vi "LEBITplc.ProcCases.vi"(0 "i ref in":refnum<vi>, 1 "selector":string, 2 "Data":T1, 3 "call cluster":T2={"Object"="", "Selector"="", "CallType"=enum."synchronous", "Async Object"="", "Async Selector"="", "Data Descriptor"="", "Data"=[], "Error #"=0, "Expire"=0}, 5 "error in (no error)":errorcluster) -> (14 "i ref out":refnum<vi>, 17 "answer cluster":T2={"Object"="", "Selector"="", "CallType"=enum."synchronous", "Async Object"="", "Async Selector"="", "Data Descriptor"="", "Data"=[], "Error #"=0, "Expire"=0}, 19 "error out":errorcluster)   [LabVIEW 2014, in "LEBITplc.lvlib"]
doc: "This method is called by a process from within the default case in the event loop. The methods of a class that are linked to events will be called from THIS method. Add your code here."
uses:
  LEBITplc.lvlib
  CS_Core/CSSystem/CoreDefs/CoreDefs.call_type.ctl
  CS_Core/BaseProcess/BaseProcess.descriptor string definition.ctl
  CS_Core/CSSystem/CoreDefs/CoreDefs.rawDataType.ctl
  CS_Core/CSSystem/CoreDefs/CoreDefs.error_severity.ctl
  CS_Core/CSSystem/CoreDefs/CoreDefs.error_type.ctl
  CS_Core/CSSystem/CoreLib/CoreLib.byte array 2 short.vi
  CS_Core/CSSystem/CoreLib/CoreLib.byte array 2 double.vi
  CS_Core/CSSystem/CoreLib/CoreLib.byte array 2 string.vi
  CS_Core/CSSystem/CoreLib/CoreLib.string 2 byte array.vi
  CS_Core/BaseProcess/BaseProcess.lvlib
  CS_Core/CSSystem/CoreLib/CoreLib.lvlib
  CS_Core/CAEObj/CAEObj.lvlib
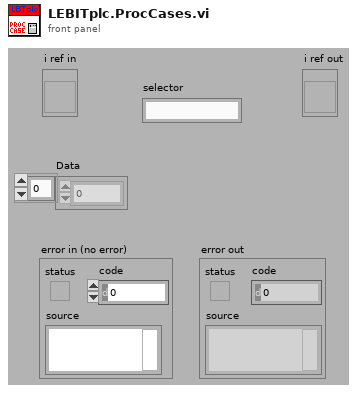
[diagram p1: front panel]
types:
  T1 = typedef "CoreDefs.rawDataType.ctl" = i8[]
  T2 = typedef "CoreDefs.call_type.ctl" = cluster{"Object":string, "Selector":string, "CallType":enum16{"simple", "synchronous", "asynchronous"}, "Async Object":string, "Async Selector":string, "Data Descriptor":T3, "Data":T1, "Error #":i32, "Expire":u32}
  T3 = typedef "BaseProcess.lvlib/BaseProcess.descriptor string definition.ctl" = string
  T4 = typedef "CoreDefs.error_type.ctl" = enum16{"no error", "can't load process", "can't unload process", "process does not exist", "can't install process", "can't remove process", "unknown function", "time out", "can't execute function", "duplicate queue name", "super not found", "caller queue invalid", "can't ping process", "unknown error", "VISA Error", "VISA timeout", "GPIB timeout", "GPIB error", "communication error", "data type mismatch", "can't read data from OPC server", "can't write data to OPC server", "OET error", "function not implemented", "process already exists", "invalid Shared Variable name", "error writing Shared Variable", "error reading Shared Variable", "invalid client name", "corrupt database", "unknown class", "call not authorized", "parameter out of range", "OET timeout: can't get data to modify", "invalid queue name", "requested operation incompatible with current state", "event undefined", "event disabled", "state undefined", "caller is not a friend", "EventBuilder: bad eventID", "EventBuilder: no DAQ devices", "a thread must not stop itself", "UNUSED ELEMENT4", "DiscArchiver: eventData incomplete", "DiscArchiver: eventData does not belong to run", "DiscArchiver: can't open file", "DiscArchiver: can't write to file", "DiscArchiver: available disc space low", "can't acquire semaphore", "error reading data from database", "notifier object is not existing", "can't register process", "can't unregister process", "illegal event type", "object disabled", "object already exists", "can't change state", "Instrument not found", "no connection to remote node", "invalid reference", "N/A", "UNUSED ELEMENT 1", "element not found", "illegal TCP/IP connection detected", "object does not exist", "invalid access ID", "unknown CS system", "invalid privilige", "unsupported data type", "unsupported server type", "IO server already exists", "Shared Variable already exists"}
  T5 = typedef "CoreDefs.error_severity.ctl" = enum16{"undefined", "information", "warning", "error", "fatal"}
  T6 = typedef "LEBITplc.lvlib/LEBITplc.i attribute.ctl" = cluster{"LLFLocation":string, "SetFileLocation":string, "nickNames":string[], "setValuePLCServiceID":i32[], "GUIServiceID":i32[], "monValuePLC":string[], "SetValueServiceID":i32[], "MonValueServiceID":i32[], "SetValue":dbl[][], "SetValueMin":dbl[], "SetValueMax":dbl[], "SetValueInfoServiceID":i32[], "GUINames":string[], "ListOfBases":string[], "Scale":dbl[], "Offset":dbl[], "setValuePLC":string[], "BaseName":string[], "ScaleServiceID":i32[], "OffsetServiceID":i32[], "AllPLCValues":string[], "CondSpecialArray":string[][], "CondSpecialIndex":i32[], "CondSpecialMonValue":dbl[], "RecentlyChanged":i32[], "SetFileLocationID":i32, "Dependent-Monitors":string[][], "LastLoadedFiles":string[], "IonGuideCalibLocation":string, "Monitor Dependent":string[], "Special":string[], "PLC?":bool[], "Start Date":string, "ListOfBasesServiceID":i32, "SETRA VISA resource":refnum<visa-resource-name>}
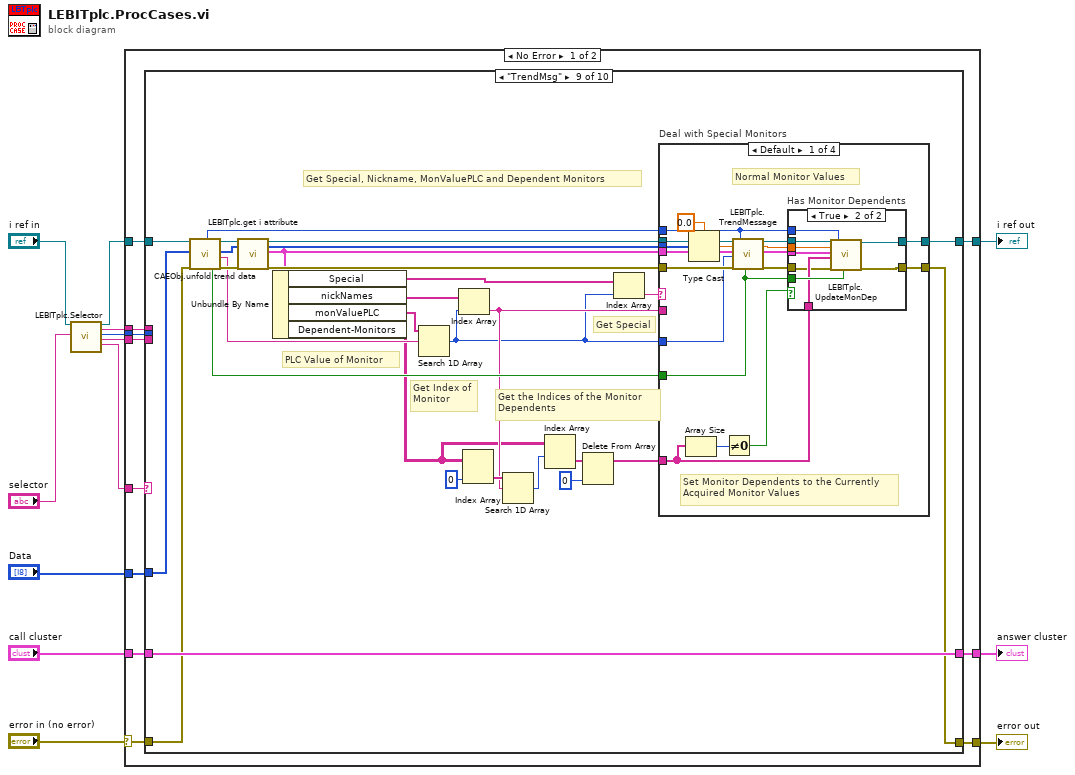
[diagram p0: block diagram]
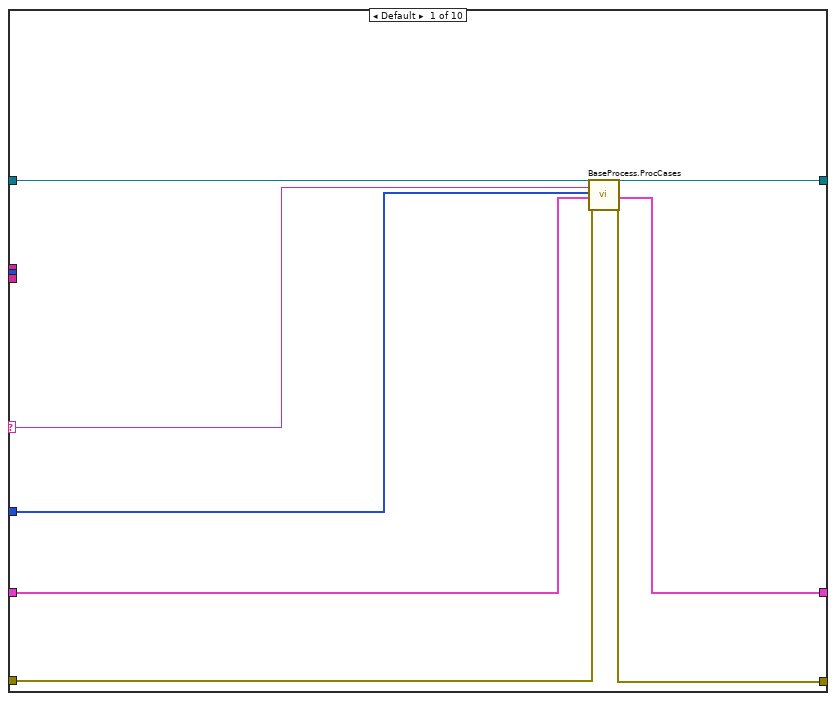
[diagram p2: hidden frame]
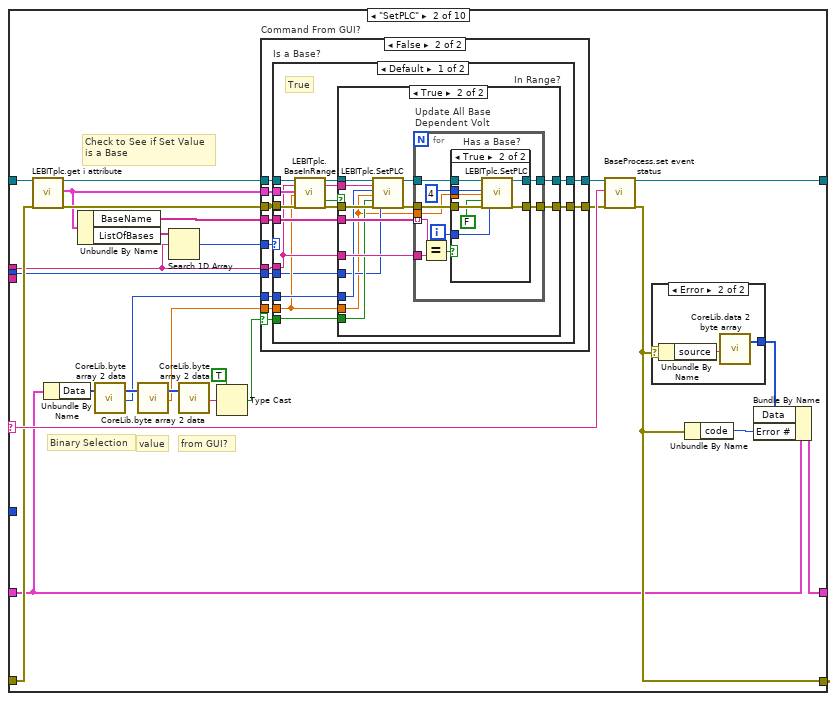
[diagram p3: hidden frame]
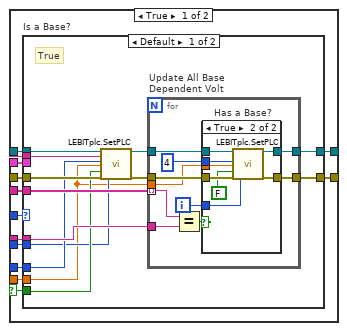
[diagram p4: hidden frame]
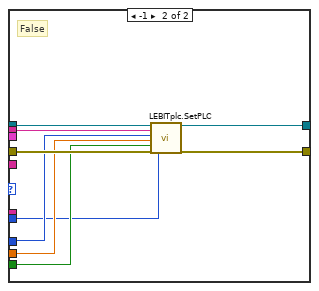
[diagram p6: hidden frame]
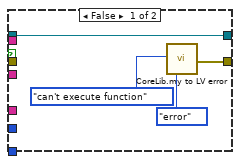
[diagram p7: hidden frame]
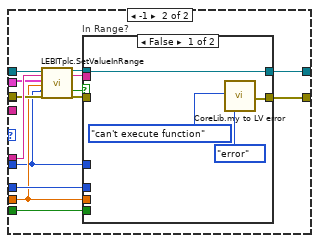
[diagram p9: hidden frame]
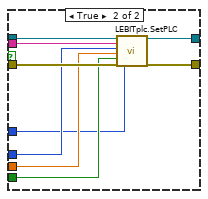
[diagram p10: hidden frame]
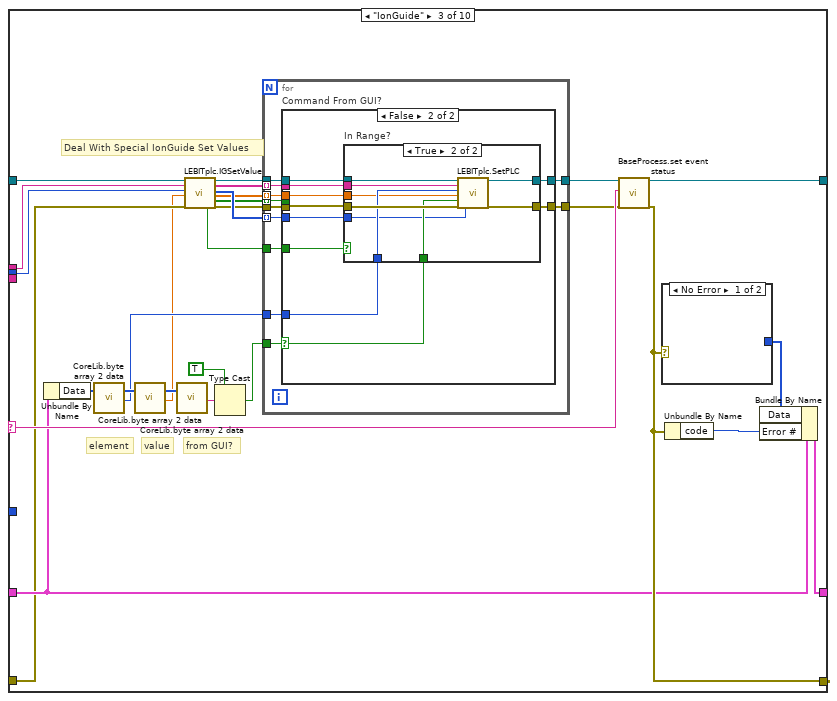
[diagram p12: hidden frame]
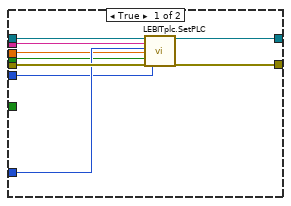
[diagram p13: hidden frame]
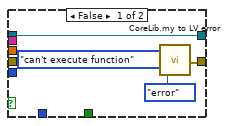
[diagram p14: hidden frame]
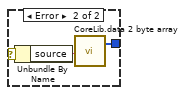
[diagram p15: hidden frame]
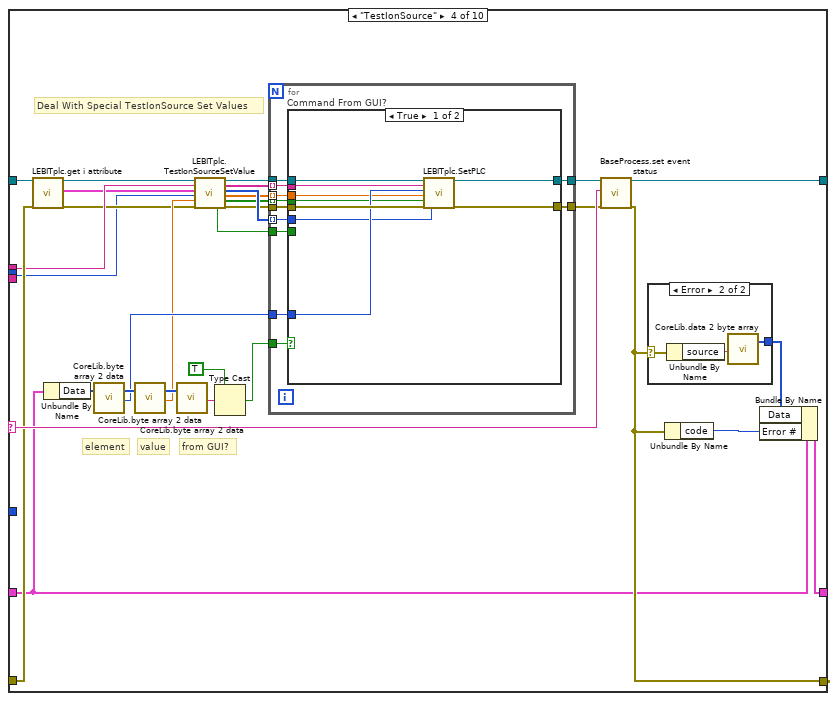
[diagram p16: hidden frame]
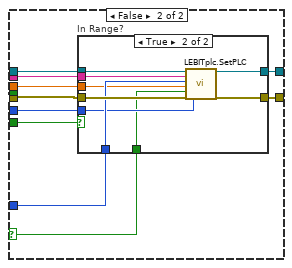
[diagram p17: hidden frame]
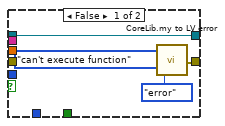
[diagram p18: hidden frame]
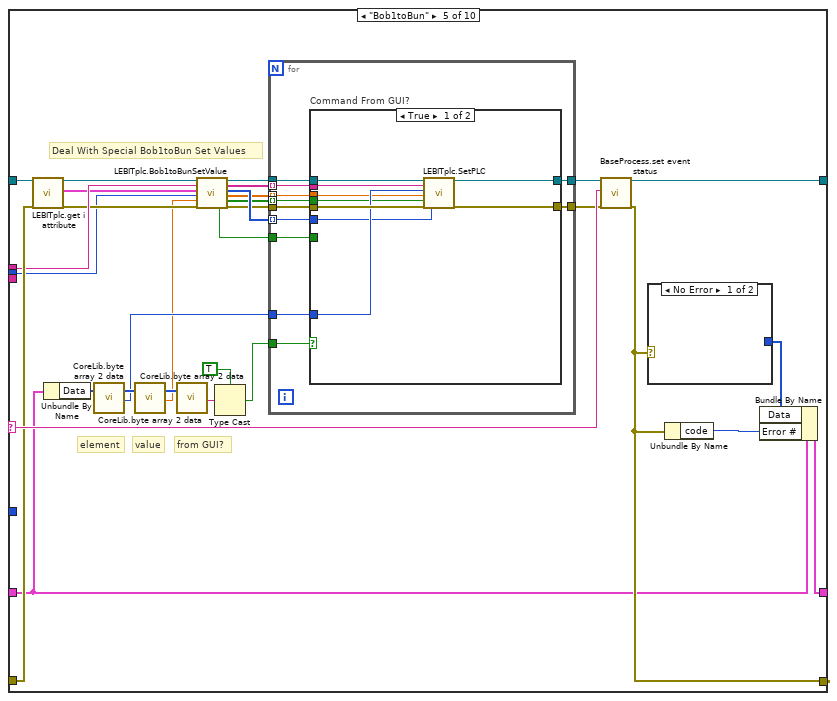
[diagram p20: hidden frame]
diagram:
  n1 = call "LEBITplc.Selector.vi"("i ref in"="i ref in", "selector in"="selector") -> ("i ref out"=w3:refnum<vi>, "Nickname"=w5:string, "index of element"=w2:i32, "Special Data"=w1:string, "selector out"=w6:string)  [unwired: 13 in]
  n2 = case shown="No Error" "error in (no error)" {
    selector: "error in (no error)" -> [w17 w808]
    tunnel: w6 -> [w24 _]
    tunnel: [w23 w809] -> w13
    tunnel: "Data" -> [w22 _]
    tunnel: "call cluster" -> [w21 w809]
    tunnel: w3 -> [w20 w810]
    tunnel: [w19 w810] -> w10
    tunnel: [w18 w808] -> w9
    tunnel: w5 -> [w16 _]
    tunnel: w2 -> [w15 _]
    tunnel: w1 -> [w14 _]
    frame No Error {
      n3 = case shown="\"TrendMsg\"" w24 {
        selector: w24 -> [w26 w54 w230 w307 w384 w460 w527 w598 _ _]
        tunnel: w22 -> [w27 _ _ _ _ _ _ _ w677 _]
        tunnel: w20 -> [w25 w51 w215 w304 w381 w457 w513 w595 w676 w793]
        tunnel: [w32 w55 w231 w308 w385 w461 w528 w599 w666 w798] -> w19
        tunnel: w21 -> [w28 w44 w229 w302 w379 w455 w524 w593 w674 w802]
        tunnel: [w29 w58 w234 w311 w388 w464 w531 w602 w674 w803] -> w23
        tunnel: w17 -> [w31 w50 w213 w303 w380 w456 w510 w594 w673 w799]
        tunnel: [w30 w56 w232 w309 w386 w462 w529 w600 w667 w797] -> w18
        tunnel: w16 -> [_ w47 w221 w294 w371 w447 w516 w585 _ _]
        tunnel: w15 -> [_ w33 w220 w282 w363 w440 w508 w573 _ _]
        tunnel: w14 -> [_ _ _ _ _ _ w509 _ _ _]
        frame Default {
          # "In the default case, always call the ProcCase method of the parent class"
          n4 = call "BaseProcess.ProcCases.vi"("i ref in"=w25, "selector"=w26, "Data"=w27, "call cluster"=w28, "error in (no error)"=w31) -> ("i ref out"=w32:refnum<vi>, "answer cluster"=w29:T2, "error out"=w30:errorcluster)  [unwired: 12 in]
        }
        frame "SetPLC" {
          # "from GUI?"
          # "value"
          # "Binary Selection"
          # "Check to See if Set Value\nis a Base"
          n5 = call "LEBITplc.get i attribute.vi"("i ref in"=w51, "error in (no error)"=w50) -> ("i ref out"=w46:refnum<vi>, "i attribute"=w43:T6, "error out"=w45:errorcluster)  [unwired: 15 in]
          n6 = Unbundle By Name(w44) -> ("Data"=w41:T1)
          n7 = Unbundle By Name(w43) -> ("BaseName"=w42:string[], "ListOfBases"=w48:string[])
          n8 = call-poly "CoreLib.byte array 2 data.vi"("byteArray"=w41) -> ("byteArray out"=w37:T1, "i16"=w35:i16)  [unwired: 16 in, 1 out]
          n9 = call-poly "CoreLib.byte array 2 data.vi"("byteArray"=w37) -> ("byteArray out"=w36:T1, "d64"=w34:dbl)  [unwired: 16 in, 1 out]
          n10 = Search 1D Array(1D array=w48, element=w47) -> (index of element=w49:i32)  [unwired: 1 in]
          n11 = call-poly "CoreLib.byte array 2 data.vi"("byteArray"=w36) -> ("string"=w39:string)  [unwired: 16 in, 2 out]
          n12 = Type Cast(type=TRUE, x=w39) -> (*(type *) &x=w38:bool)
          n13 = case "Command From GUI?" shown="False" w38 {
            selector: w38 -> [w63 w117]
            tunnel: [w71 w125] -> w53
            tunnel: [w70 w124] -> w52
            tunnel: w49 -> [w69 w123]
            tunnel: w47 -> [w68 w122]
            tunnel: w46 -> [w67 w121]
            tunnel: w45 -> [w66 w118]
            tunnel: w43 -> [w65 w120]
            tunnel: w42 -> [w64 w119]
            tunnel: w35 -> [w62 w115]
            tunnel: w34 -> [w61 w116]
            tunnel: w33 -> [w60 w114]
            frame True {
              n14 = case "Is a Base?" shown="Default" w69 {
                tunnel: w67 -> [w80 w110]
                tunnel: [w82 w113] -> w71
                tunnel: [w83 w112] -> w70
                tunnel: w66 -> [w78 w111]
                tunnel: w68 -> [w84 _]
                tunnel: w64 -> [w81 _]
                tunnel: w68 -> [w79 w109]
                tunnel: w65 -> [_ _]
                tunnel: w63 -> [w75 w106]
                tunnel: w62 -> [w74 w108]
                tunnel: w61 -> [w72 w107]
                tunnel: w60 -> [w73 w105]
                frame Default {
                  # "True"
                  n15 = call "LEBITplc.SetPLC.vi"("i ref in"=w80, "CommandName"=w79, "Binary Selection"=w74, "Value"=w72, "log?"=w75, "error IO"=w78, "index of element"=w73) -> ("i ref out"=w77:refnum<vi>, "error out"=w76:errorcluster)  [unwired: 11 in]
                  n16 = for "Update All Base \nDependent Volt" {
                    tunnel: w84 -> [w94]
                    tunnel: w77 -> [w92]
                    tunnel: w76 -> [w91]
                    tunnel: [w90] -> w83
                    tunnel: [w89] -> w82
                    tunnel: w81 -> [w88] mode=indexing
                    tunnel: w72 -> [w86]
                    i -> [w87]
                    n17 = Equal?(x=w88, y=w94) -> (x = y?=w93:bool)
                    n18 = case "Has a Base?" shown="True" w93 {
                      tunnel: w92 -> [w95 w102]
                      tunnel: w91 -> [w96 w101]
                      tunnel: [w96 w103] -> w90
                      tunnel: [w95 w104] -> w89
                      tunnel: w87 -> [_ w99]
                      tunnel: w86 -> [_ w98]
                      tunnel: i16 4 ("Binary Selection") -> [_ w97]
                      frame False {
                      }
                      frame True {
                        n19 = call "LEBITplc.SetPLC.vi"("i ref in"=w102, "Binary Selection"=w97, "Value"=w98, "log?"=FALSE, "error IO"=w101, "index of element"=w99) -> ("i ref out"=w104:refnum<vi>, "error out"=w103:errorcluster)  [unwired: 12 in]
                      }
                    }
                  }
                }
                frame -1 {
                  # "False"
                  n20 = call "LEBITplc.SetPLC.vi"("i ref in"=w110, "CommandName"=w109, "Binary Selection"=w108, "Value"=w107, "log?"=w106, "error IO"=w111, "index of element"=w105) -> ("i ref out"=w113:refnum<vi>, "error out"=w112:errorcluster)  [unwired: 11 in]
                }
              }
            }
            frame False {
              n21 = case "Is a Base?" shown="Default" w123 {
                tunnel: w121 -> [w135 w189]
                tunnel: [w139 w191] -> w125
                tunnel: [w140 w190] -> w124
                tunnel: w118 -> [w134 _]
                tunnel: w122 -> [w130 w187]
                tunnel: w119 -> [w138 _]
                tunnel: w120 -> [w133 w182]
                tunnel: w118 -> [_ w186]
                tunnel: w117 -> [w127 w180]
                tunnel: w116 -> [w128 w179]
                tunnel: w115 -> [w129 w181]
                tunnel: w114 -> [w126 w178]
                frame Default {
                  # "True"
                  n22 = call "LEBITplc.BaseInRange.vi"("i ref in"=w135, "CommandName in"=w130, "i attribute in"=w133, "value"=w128, "error out in"=w134) -> ("i ref out"=w137:refnum<vi>, "CommandName out"=w131:string, "In Range?"=w132:bool, "error out"=w136:errorcluster)  [unwired: 11 in]
                  n23 = case "In Range?" shown="True" w132 {
                    tunnel: w130 -> [_ w157]
                    tunnel: [w142 w156] -> w140
                    tunnel: [w141 w155] -> w139
                    tunnel: w138 -> [_ w154]
                    tunnel: w137 -> [w141 w151]
                    tunnel: w136 -> [_ w150]
                    tunnel: w131 -> [_ w149]
                    tunnel: w129 -> [_ w148]
                    tunnel: w128 -> [_ w145]
                    tunnel: w127 -> [_ w147]
                    tunnel: w126 -> [_ w146]
                    frame False {
                      n24 = call "CoreLib.my to LV error.vi"("ErrorTypes"=CoreDefs.error_type."can't execute function", "severityLevel"=CoreDefs.error_severity."error") -> ("myErrorCluster"=w142:errorcluster)  [unwired: 16 in, 1 out]
                    }
                    frame True {
                      n25 = call "LEBITplc.SetPLC.vi"("i ref in"=w151, "CommandName"=w149, "Binary Selection"=w148, "Value"=w145, "log?"=w147, "error IO"=w150, "index of element"=w146) -> ("i ref out"=w153:refnum<vi>, "error out"=w152:errorcluster)  [unwired: 11 in]
                      n26 = for "Update All Base \nDependent Volt" {
                        tunnel: w157 -> [w167]
                        tunnel: w153 -> [w162]
                        tunnel: w152 -> [w163]
                        tunnel: [w164] -> w156
                        tunnel: [w165] -> w155
                        tunnel: w154 -> [w166] mode=indexing
                        tunnel: w145 -> [w160]
                        i -> [w161]
                        n27 = Equal?(x=w166, y=w167) -> (x = y?=w158:bool)
                        n28 = case "Has a Base?" shown="True" w158 {
                          tunnel: w162 -> [w168 w175]
                          tunnel: w163 -> [w169 w174]
                          tunnel: [w169 w176] -> w164
                          tunnel: [w168 w177] -> w165
                          tunnel: w161 -> [_ w172]
                          tunnel: w160 -> [_ w171]
                          tunnel: i16 4 ("Binary Selection") -> [_ w170]
                          frame False {
                          }
                          frame True {
                            n29 = call "LEBITplc.SetPLC.vi"("i ref in"=w175, "Binary Selection"=w170, "Value"=w171, "log?"=FALSE, "error IO"=w174, "index of element"=w172) -> ("i ref out"=w177:refnum<vi>, "error out"=w176:errorcluster)  [unwired: 12 in]
                          }
                        }
                      }
                    }
                  }
                }
                frame -1 {
                  n30 = call "LEBITplc.SetValueInRange.vi"("i ref in"=w189, "CommandName in"=w187, "i attribute in"=w182, "value in"=w179, "index of element"=w178, "error out in"=w186) -> ("i ref out"=w188:refnum<vi>, "CommandName out"=w185:string, "In Range?"=w183:bool, "error out"=w184:errorcluster)  [unwired: 9 in, 1 out]
                  n31 = case "In Range?" shown="False" w183 {
                    tunnel: [w194 w204] -> w191
                    tunnel: [w195 w203] -> w190
                    tunnel: w184 -> [_ w202]
                    tunnel: w188 -> [w194 w201]
                    tunnel: w185 -> [_ w200]
                    tunnel: w181 -> [_ w199]
                    tunnel: w180 -> [_ w198]
                    tunnel: w179 -> [_ w197]
                    tunnel: w178 -> [_ w196]
                    frame False {
                      n32 = call "CoreLib.my to LV error.vi"("ErrorTypes"=CoreDefs.error_type."can't execute function", "severityLevel"=CoreDefs.error_severity."error") -> ("myErrorCluster"=w195:errorcluster)  [unwired: 16 in, 1 out]
                    }
                    frame True {
                      n33 = call "LEBITplc.SetPLC.vi"("i ref in"=w201, "CommandName"=w200, "Binary Selection"=w199, "Value"=w197, "log?"=w198, "error IO"=w202, "index of element"=w196) -> ("i ref out"=w204:refnum<vi>, "error out"=w203:errorcluster)  [unwired: 11 in]
                    }
                  }
                }
              }
            }
          }
          n34 = call "BaseProcess.set event status.vi"("i ref in"=w53, "EventStatus"=w54, "error in (no error)"=w52) -> ("i ref out"=w55:refnum<vi>, "error out"=w56:errorcluster)  [unwired: 14 in, 1 out]
          n35 = case shown="Error" w56 {
            selector: w56 -> [_ w207]
            tunnel: [_ w206] -> w57
            frame No Error {
            }
            frame Error {
              n36 = Unbundle By Name(w207) -> ("source"=w205:string)
              n37 = call-poly "CoreLib.data 2 byte array.vi"("string"=w205) -> ("byteArray out"=w206:T1)  [unwired: 18 in]
            }
          }
          n38 = Unbundle By Name(w56) -> ("code"=w59:i32)
          n39 = Bundle By Name(cluster=w44, "Data"=w57, "Error #"=w59) -> (w58:T2)
        }
        frame "IonGuide" {
          # "from GUI?"
          # "value"
          # "element"
          # "Deal With Special IonGuide Set Values"
          n40 = Unbundle By Name(w229) -> ("Data"=w225:T1)
          n41 = call-poly "CoreLib.byte array 2 data.vi"("byteArray"=w225) -> ("byteArray out"=w224:T1, "i16"=w222:i16)  [unwired: 16 in, 1 out]
          n42 = call-poly "CoreLib.byte array 2 data.vi"("byteArray"=w224) -> ("byteArray out"=w223:T1, "d64"=w208:dbl)  [unwired: 16 in, 1 out]
          n43 = call-poly "CoreLib.byte array 2 data.vi"("byteArray"=w223) -> ("string"=w227:string)  [unwired: 16 in, 2 out]
          n44 = call "LEBITplc.IGSetValue.vi"("i ref in"=w215, "Nickname in"=w221, "index in"=w220, "value"=w208, "error in (no error)"=w213) -> ("In Range?"=w209:bool, "i ref out"=w214:refnum<vi>, "Nicknames out"=w219:string[], "Index out"=w218:i32[], "values"=w212:dbl[], "Log out"=w211:bool[], "error out"=w210:errorcluster)  [unwired: 8 in]
          n45 = Type Cast(type=TRUE, x=w227) -> (*(type *) &x=w226:bool)
          n46 = for {
            tunnel: [w246] -> w217
            tunnel: [w245] -> w216
            tunnel: w214 -> [w244]
            tunnel: w210 -> [w243]
            tunnel: w226 -> [w242]
            tunnel: w222 -> [w241]
            tunnel: w219 -> [w240] mode=indexing
            tunnel: w211 -> [w239] mode=indexing
            tunnel: w218 -> [w238] mode=indexing
            tunnel: w212 -> [w237] mode=indexing
            tunnel: w209 -> [w236]
            n47 = case "Command From GUI?" shown="False" w242 {
              selector: w242 -> [_ w263]
              tunnel: [w255 w265] -> w246
              tunnel: [w254 w264] -> w245
              tunnel: w240 -> [w253 w259]
              tunnel: w244 -> [w252 w260]
              tunnel: w243 -> [w251 w258]
              tunnel: w241 -> [w250 w262]
              tunnel: w239 -> [w247 _]
              tunnel: w238 -> [w249 w261]
              tunnel: w237 -> [w248 w257]
              tunnel: w236 -> [_ w256]
              frame True {
                n48 = call "LEBITplc.SetPLC.vi"("i ref in"=w252, "CommandName"=w253, "Binary Selection"=w250, "Value"=w248, "log?"=w247, "error IO"=w251, "index of element"=w249) -> ("i ref out"=w255:refnum<vi>, "error out"=w254:errorcluster)  [unwired: 11 in]
              }
              frame False {
                n49 = case "In Range?" shown="True" w256 {
                  tunnel: [w268 w278] -> w265
                  tunnel: [w269 w277] -> w264
                  tunnel: w258 -> [_ w276]
                  tunnel: w260 -> [w268 w275]
                  tunnel: w259 -> [_ w274]
                  tunnel: w263 -> [_ w272]
                  tunnel: w262 -> [_ w273]
                  tunnel: w261 -> [_ w271]
                  tunnel: w257 -> [_ w270]
                  frame False {
                    n50 = call "CoreLib.my to LV error.vi"("ErrorTypes"=CoreDefs.error_type."can't execute function", "severityLevel"=CoreDefs.error_severity."error") -> ("myErrorCluster"=w269:errorcluster)  [unwired: 16 in, 1 out]
                  }
                  frame True {
                    n51 = call "LEBITplc.SetPLC.vi"("i ref in"=w275, "CommandName"=w274, "Binary Selection"=w273, "Value"=w270, "log?"=w272, "error IO"=w276, "index of element"=w271) -> ("i ref out"=w278:refnum<vi>, "error out"=w277:errorcluster)  [unwired: 11 in]
                  }
                }
              }
            }
          }
          n52 = call "BaseProcess.set event status.vi"("i ref in"=w217, "EventStatus"=w230, "error in (no error)"=w216) -> ("i ref out"=w231:refnum<vi>, "error out"=w232:errorcluster)  [unwired: 14 in, 1 out]
          n53 = case shown="No Error" w232 {
            selector: w232 -> [_ w281]
            tunnel: [_ w280] -> w233
            frame No Error {
            }
            frame Error {
              n54 = Unbundle By Name(w281) -> ("source"=w279:string)
              n55 = call-poly "CoreLib.data 2 byte array.vi"("string"=w279) -> ("byteArray out"=w280:T1)  [unwired: 18 in]
            }
          }
          n56 = Unbundle By Name(w232) -> ("code"=w235:i32)
          n57 = Bundle By Name(cluster=w229, "Data"=w233, "Error #"=w235) -> (w234:T2)
        }
        frame "TestIonSource" {
          # "from GUI?"
          # "value"
          # "element"
          # "Deal With Special TestIonSource Set Values"
          n58 = call "LEBITplc.get i attribute.vi"("i ref in"=w304, "error in (no error)"=w303) -> ("i ref out"=w286:refnum<vi>, "i attribute"=w284:T6, "error out"=w288:errorcluster)  [unwired: 15 in]
          n59 = Unbundle By Name(w302) -> ("Data"=w298:T1)
          n60 = call-poly "CoreLib.byte array 2 data.vi"("byteArray"=w298) -> ("byteArray out"=w297:T1, "i16"=w295:i16)  [unwired: 16 in, 1 out]
          n61 = call-poly "CoreLib.byte array 2 data.vi"("byteArray"=w297) -> ("byteArray out"=w296:T1, "d64"=w289:dbl)  [unwired: 16 in, 1 out]
          n62 = call-poly "CoreLib.byte array 2 data.vi"("byteArray"=w296) -> ("string"=w300:string)  [unwired: 16 in, 2 out]
          n63 = call "LEBITplc.TestIonSourceSetValue.vi"("i ref in"=w286, "Nickname in"=w294, "i attribute in"=w284, "index in"=w282, "value"=w289, "error in"=w288) -> ("In Range?"=w283:bool, "i ref out"=w285:refnum<vi>, "Nicknames out"=w293:string[], "Index out"=w292:i32[], "values"=w291:dbl[], "Log Out"=w290:bool[], "error out"=w287:errorcluster)  [unwired: 7 in]
          n64 = Type Cast(type=TRUE, x=w300) -> (*(type *) &x=w299:bool)
          n65 = for {
            tunnel: [w323] -> w306
            tunnel: [w322] -> w305
            tunnel: w285 -> [w321]
            tunnel: w287 -> [w320]
            tunnel: w299 -> [w319]
            tunnel: w295 -> [w318]
            tunnel: w293 -> [w317] mode=indexing
            tunnel: w290 -> [w316] mode=indexing
            tunnel: w292 -> [w315] mode=indexing
            tunnel: w291 -> [w314] mode=indexing
            tunnel: w283 -> [w313]
            n66 = case "Command From GUI?" shown="True" w319 {
              selector: w319 -> [_ w333]
              tunnel: [w332 w342] -> w323
              tunnel: [w331 w341] -> w322
              tunnel: w317 -> [w330 w337]
              tunnel: w321 -> [w329 w338]
              tunnel: w320 -> [w328 w336]
              tunnel: w318 -> [w327 w340]
              tunnel: w316 -> [w324 _]
              tunnel: w315 -> [w326 w339]
              tunnel: w314 -> [w325 w335]
              tunnel: w313 -> [_ w334]
              frame True {
                n67 = call "LEBITplc.SetPLC.vi"("i ref in"=w329, "CommandName"=w330, "Binary Selection"=w327, "Value"=w325, "log?"=w324, "error IO"=w328, "index of element"=w326) -> ("i ref out"=w332:refnum<vi>, "error out"=w331:errorcluster)  [unwired: 11 in]
              }
              frame False {
                n68 = case "In Range?" shown="True" w334 {
                  tunnel: [w345 w355] -> w342
                  tunnel: [w346 w354] -> w341
                  tunnel: w336 -> [_ w353]
                  tunnel: w338 -> [w345 w352]
                  tunnel: w337 -> [_ w351]
                  tunnel: w340 -> [_ w350]
                  tunnel: w339 -> [_ w349]
                  tunnel: w335 -> [_ w348]
                  tunnel: w333 -> [_ w347]
                  frame False {
                    n69 = call "CoreLib.my to LV error.vi"("ErrorTypes"=CoreDefs.error_type."can't execute function", "severityLevel"=CoreDefs.error_severity."error") -> ("myErrorCluster"=w346:errorcluster)  [unwired: 16 in, 1 out]
                  }
                  frame True {
                    n70 = call "LEBITplc.SetPLC.vi"("i ref in"=w352, "CommandName"=w351, "Binary Selection"=w350, "Value"=w348, "log?"=w347, "error IO"=w353, "index of element"=w349) -> ("i ref out"=w355:refnum<vi>, "error out"=w354:errorcluster)  [unwired: 11 in]
                  }
                }
              }
            }
          }
          n71 = call "BaseProcess.set event status.vi"("i ref in"=w306, "EventStatus"=w307, "error in (no error)"=w305) -> ("i ref out"=w308:refnum<vi>, "error out"=w309:errorcluster)  [unwired: 14 in, 1 out]
          n72 = case shown="Error" w309 {
            selector: w309 -> [_ w358]
            tunnel: [_ w357] -> w310
            frame No Error {
            }
            frame Error {
              n73 = Unbundle By Name(w358) -> ("source"=w356:string)
              n74 = call-poly "CoreLib.data 2 byte array.vi"("string"=w356) -> ("byteArray out"=w357:T1)  [unwired: 18 in]
            }
          }
          n75 = Unbundle By Name(w309) -> ("code"=w312:i32)
          n76 = Bundle By Name(cluster=w302, "Data"=w310, "Error #"=w312) -> (w311:T2)
        }
        frame "Bob1toBun" {
          # "from GUI?"
          # "value"
          # "element"
          # "Deal With Special Bob1toBun Set Values"
          n77 = call "LEBITplc.get i attribute.vi"("i ref in"=w381, "error in (no error)"=w380) -> ("i ref out"=w368:refnum<vi>, "i attribute"=w364:T6, "error out"=w365:errorcluster)  [unwired: 15 in]
          n78 = Unbundle By Name(w379) -> ("Data"=w375:T1)
          n79 = call-poly "CoreLib.byte array 2 data.vi"("byteArray"=w375) -> ("byteArray out"=w374:T1, "i16"=w372:i16)  [unwired: 16 in, 1 out]
          n80 = call-poly "CoreLib.byte array 2 data.vi"("byteArray"=w374) -> ("byteArray out"=w373:T1, "d64"=w362:dbl)  [unwired: 16 in, 1 out]
          n81 = call-poly "CoreLib.byte array 2 data.vi"("byteArray"=w373) -> ("string"=w377:string)  [unwired: 16 in, 2 out]
          n82 = call "LEBITplc.Bob1toBunSetValue.vi"("i ref in"=w368, "Nickname in"=w371, "i attribute in"=w364, "index in"=w363, "value"=w362, "error in"=w365) -> ("In Range?"=w360:bool, "i ref out"=w367:refnum<vi>, "Nicknames out"=w370:string[], "Index out"=w369:i32[], "values"=w361:dbl[], "Log Out?"=w359:bool[], "error out"=w366:errorcluster)  [unwired: 7 in]
          n83 = Type Cast(type=TRUE, x=w377) -> (*(type *) &x=w376:bool)
          n84 = for {
            tunnel: [w400] -> w383
            tunnel: [w399] -> w382
            tunnel: w367 -> [w398]
            tunnel: w366 -> [w397]
            tunnel: w376 -> [w396]
            tunnel: w372 -> [w395]
            tunnel: w370 -> [w394] mode=indexing
            tunnel: w369 -> [w393] mode=indexing
            tunnel: w361 -> [w392] mode=indexing
            tunnel: w360 -> [w391]
            tunnel: w359 -> [w390] mode=indexing
            n85 = case "Command From GUI?" shown="True" w396 {
              selector: w396 -> [_ w417]
              tunnel: [w409 w419] -> w400
              tunnel: [w408 w418] -> w399
              tunnel: w394 -> [w407 w414]
              tunnel: w398 -> [w406 w412]
              tunnel: w397 -> [w405 w413]
              tunnel: w395 -> [w404 w416]
              tunnel: w393 -> [w403 w415]
              tunnel: w392 -> [w402 w411]
              tunnel: w391 -> [_ w410]
              tunnel: w390 -> [w401 _]
              frame True {
                n86 = call "LEBITplc.SetPLC.vi"("i ref in"=w406, "CommandName"=w407, "Binary Selection"=w404, "Value"=w402, "log?"=w401, "error IO"=w405, "index of element"=w403) -> ("i ref out"=w409:refnum<vi>, "error out"=w408:errorcluster)  [unwired: 11 in]
              }
              frame False {
                n87 = case "In Range?" shown="True" w410 {
                  tunnel: [w422 w432] -> w419
                  tunnel: [w423 w431] -> w418
                  tunnel: w413 -> [_ w430]
                  tunnel: w412 -> [w422 w429]
                  tunnel: w414 -> [_ w428]
                  tunnel: w417 -> [_ w426]
                  tunnel: w416 -> [_ w427]
                  tunnel: w415 -> [_ w425]
                  tunnel: w411 -> [_ w424]
                  frame False {
                    n88 = call "CoreLib.my to LV error.vi"("ErrorTypes"=CoreDefs.error_type."can't execute function", "severityLevel"=CoreDefs.error_severity."error") -> ("myErrorCluster"=w423:errorcluster)  [unwired: 16 in, 1 out]
                  }
                  frame True {
                    n89 = call "LEBITplc.SetPLC.vi"("i ref in"=w429, "CommandName"=w428, "Binary Selection"=w427, "Value"=w424, "log?"=w426, "error IO"=w430, "index of element"=w425) -> ("i ref out"=w432:refnum<vi>, "error out"=w431:errorcluster)  [unwired: 11 in]
                  }
                }
              }
            }
          }
          n90 = call "BaseProcess.set event status.vi"("i ref in"=w383, "EventStatus"=w384, "error in (no error)"=w382) -> ("i ref out"=w385:refnum<vi>, "error out"=w386:errorcluster)  [unwired: 14 in, 1 out]
          n91 = case shown="No Error" w386 {
            selector: w386 -> [_ w435]
            tunnel: [_ w434] -> w387
            frame No Error {
            }
            frame Error {
              n92 = Unbundle By Name(w435) -> ("source"=w433:string)
              n93 = call-poly "CoreLib.data 2 byte array.vi"("string"=w433) -> ("byteArray out"=w434:T1)  [unwired: 18 in]
            }
          }
          n94 = Unbundle By Name(w386) -> ("code"=w389:i32)
          n95 = Bundle By Name(cluster=w379, "Data"=w387, "Error #"=w389) -> (w388:T2)
        }
        frame "PressureSafety" {
          # "from GUI?"
          # "value"
          # "element"
          # "Make sure it is safe to change \npercent neon"
          n96 = call "LEBITplc.get i attribute.vi"("i ref in"=w457, "error in (no error)"=w456) -> ("i ref out"=w444:refnum<vi>, "i attribute"=w442:T6, "error out"=w446:errorcluster)  [unwired: 15 in]
          n97 = Unbundle By Name(w455) -> ("Data"=w454:T1)
          n98 = call-poly "CoreLib.byte array 2 data.vi"("byteArray"=w454) -> ("byteArray out"=w450:T1, "i16"=w436:i16)  [unwired: 16 in, 1 out]
          n99 = call-poly "CoreLib.byte array 2 data.vi"("byteArray"=w450) -> ("byteArray out"=w449:T1, "d64"=w437:dbl)  [unwired: 16 in, 1 out]
          n100 = call-poly "CoreLib.byte array 2 data.vi"("byteArray"=w449) -> ("string"=w452:string)  [unwired: 16 in, 2 out]
          n101 = call "LEBITplc.PressureSafety.vi"("i ref in"=w444, "Nickname in"=w447, "i attribute in"=w442, "value"=w437, "index in"=w440, "error in"=w446) -> ("i ref out"=w443:refnum<vi>, "Nickname out"=w448:string, "i attribute out"=w441:T6, "value out"=w439:dbl, "index out"=w438:i32, "error out"=w445:errorcluster)  [unwired: 8 in]
          n102 = Type Cast(type=TRUE, x=w452) -> (*(type *) &x=w451:bool)
          n103 = case "Command From GUI?" shown="False" w451 {
            selector: w451 -> [w469 w483]
            tunnel: [w474 w489] -> w459
            tunnel: [w473 w488] -> w458
            tunnel: w448 -> [w472 w487]
            tunnel: w443 -> [w471 w486]
            tunnel: w445 -> [w470 w484]
            tunnel: w441 -> [_ w485]
            tunnel: w439 -> [w467 w476]
            tunnel: w436 -> [w466 w475]
            tunnel: w438 -> [w468 w478]
            frame True {
              n104 = call "LEBITplc.SetPLC.vi"("i ref in"=w471, "CommandName"=w472, "Binary Selection"=w466, "Value"=w467, "log?"=w469, "error IO"=w470, "index of element"=w468) -> ("i ref out"=w474:refnum<vi>, "error out"=w473:errorcluster)  [unwired: 11 in]
            }
            frame False {
              n105 = call "LEBITplc.SetValueInRange.vi"("i ref in"=w486, "CommandName in"=w487, "i attribute in"=w485, "value in"=w476, "index of element"=w478, "error out in"=w484) -> ("i ref out"=w482:refnum<vi>, "CommandName out"=w481:string, "value out"=w477:dbl, "In Range?"=w479:bool, "error out"=w480:errorcluster)  [unwired: 9 in]
              n106 = case "In Range?" shown="True" w479 {
                tunnel: [w492 w502] -> w489
                tunnel: [w493 w501] -> w488
                tunnel: w480 -> [_ w500]
                tunnel: w482 -> [w492 w499]
                tunnel: w481 -> [_ w498]
                tunnel: w475 -> [_ w497]
                tunnel: w483 -> [_ w496]
                tunnel: w478 -> [_ w495]
                tunnel: w477 -> [_ w494]
                frame False {
                  n107 = call "CoreLib.my to LV error.vi"("ErrorTypes"=CoreDefs.error_type."can't execute function", "severityLevel"=CoreDefs.error_severity."error") -> ("myErrorCluster"=w493:errorcluster)  [unwired: 16 in, 1 out]
                }
                frame True {
                  n108 = call "LEBITplc.SetPLC.vi"("i ref in"=w499, "CommandName"=w498, "Binary Selection"=w497, "Value"=w494, "log?"=w496, "error IO"=w500, "index of element"=w495) -> ("i ref out"=w502:refnum<vi>, "error out"=w501:errorcluster)  [unwired: 11 in]
                }
              }
            }
          }
          n109 = call "BaseProcess.set event status.vi"("i ref in"=w459, "EventStatus"=w460, "error in (no error)"=w458) -> ("i ref out"=w461:refnum<vi>, "error out"=w462:errorcluster)  [unwired: 14 in, 1 out]
          n110 = case shown="No Error" w462 {
            selector: w462 -> [_ w505]
            tunnel: [_ w504] -> w463
            frame No Error {
            }
            frame Error {
              n111 = Unbundle By Name(w505) -> ("source"=w503:string)
              n112 = call-poly "CoreLib.data 2 byte array.vi"("string"=w503) -> ("byteArray out"=w504:T1)  [unwired: 18 in]
            }
          }
          n113 = Unbundle By Name(w462) -> ("code"=w465:i32)
          n114 = Bundle By Name(cluster=w455, "Data"=w463, "Error #"=w465) -> (w464:T2)
        }
        frame "Mosfet" {
          # "from GUI?"
          # "value"
          # "element"
          # "Deal With Mosfet Set Values"
          n115 = Unbundle By Name(w524) -> ("Data"=w520:T1)
          n116 = call-poly "CoreLib.byte array 2 data.vi"("byteArray"=w520) -> ("byteArray out"=w519:T1, "i16"=w506:i16)  [unwired: 16 in, 1 out]
          n117 = call-poly "CoreLib.byte array 2 data.vi"("byteArray"=w519) -> ("byteArray out"=w518:T1, "d64"=w507:dbl)  [unwired: 16 in, 1 out]
          n118 = call "LEBITplc.MosfetSetValue.vi"("i ref in"=w513, "index in"=w508, "Special Data in"=w509, "error in (no error)"=w510, "element"=w506, "value"=w507) -> ("i ref out"=w512:refnum<vi>, "error IO"=w511:errorcluster)  [unwired: 12 in]
          n119 = call-poly "CoreLib.byte array 2 data.vi"("byteArray"=w518) -> ("string"=w522:string)  [unwired: 16 in, 2 out]
          n120 = Type Cast(type=TRUE, x=w522) -> (*(type *) &x=w521:bool)
          n121 = call "LEBITplc.get i attribute.vi"("i ref in"=w512, "error in (no error)"=w511) -> ("i ref out"=w515:refnum<vi>, "i attribute"=w517:T6, "error out"=w514:errorcluster)  [unwired: 15 in]
          n122 = case "Command From GUI?" shown="True" w521 {
            selector: w521 -> [w536 w551]
            tunnel: [w541 w556] -> w526
            tunnel: [w540 w555] -> w525
            tunnel: w516 -> [w539 w554]
            tunnel: w515 -> [w538 w553]
            tunnel: w514 -> [w537 w546]
            tunnel: w517 -> [_ w552]
            tunnel: w507 -> [w533 w543]
            tunnel: w506 -> [w534 w542]
            tunnel: w508 -> [w535 w545]
            frame True {
              n123 = call "LEBITplc.SetPLC.vi"("i ref in"=w538, "CommandName"=w539, "Binary Selection"=w534, "Value"=w533, "log?"=w536, "error IO"=w537, "index of element"=w535) -> ("i ref out"=w541:refnum<vi>, "error out"=w540:errorcluster)  [unwired: 11 in]
            }
            frame False {
              n124 = call "LEBITplc.SetValueInRange.vi"("i ref in"=w553, "CommandName in"=w554, "i attribute in"=w552, "value in"=w543, "index of element"=w545, "error out in"=w546) -> ("i ref out"=w550:refnum<vi>, "CommandName out"=w549:string, "value out"=w544:dbl, "In Range?"=w547:bool, "error out"=w548:errorcluster)  [unwired: 9 in]
              n125 = case "In Range?" shown="True" w547 {
                tunnel: [w559 w569] -> w556
                tunnel: [w560 w568] -> w555
                tunnel: w548 -> [_ w567]
                tunnel: w550 -> [w559 w566]
                tunnel: w549 -> [_ w565]
                tunnel: w551 -> [_ w563]
                tunnel: w542 -> [_ w564]
                tunnel: w545 -> [_ w562]
                tunnel: w544 -> [_ w561]
                frame False {
                  n126 = call "CoreLib.my to LV error.vi"("ErrorTypes"=CoreDefs.error_type."can't execute function", "severityLevel"=CoreDefs.error_severity."error") -> ("myErrorCluster"=w560:errorcluster)  [unwired: 16 in, 1 out]
                }
                frame True {
                  n127 = call "LEBITplc.SetPLC.vi"("i ref in"=w566, "CommandName"=w565, "Binary Selection"=w564, "Value"=w561, "log?"=w563, "error IO"=w567, "index of element"=w562) -> ("i ref out"=w569:refnum<vi>, "error out"=w568:errorcluster)  [unwired: 11 in]
                }
              }
            }
          }
          n128 = call "BaseProcess.set event status.vi"("i ref in"=w526, "EventStatus"=w527, "error in (no error)"=w525) -> ("i ref out"=w528:refnum<vi>, "error out"=w529:errorcluster)  [unwired: 14 in, 1 out]
          n129 = case shown="No Error" w529 {
            selector: w529 -> [_ w572]
            tunnel: [_ w571] -> w530
            frame No Error {
            }
            frame Error {
              n130 = Unbundle By Name(w572) -> ("source"=w570:string)
              n131 = call-poly "CoreLib.data 2 byte array.vi"("string"=w570) -> ("byteArray out"=w571:T1)  [unwired: 18 in]
            }
          }
          n132 = Unbundle By Name(w529) -> ("code"=w532:i32)
          n133 = Bundle By Name(cluster=w524, "Data"=w530, "Error #"=w532) -> (w531:T2)
        }
        frame "Penning" {
          # "from GUI?"
          # "value"
          # "element"
          # "Deal With Special Penning Set Values"
          n134 = call "LEBITplc.get i attribute.vi"("i ref in"=w595, "error in (no error)"=w594) -> ("i ref out"=w583:refnum<vi>, "i attribute"=w579:T6, "error out"=w581:errorcluster)  [unwired: 15 in]
          n135 = Unbundle By Name(w593) -> ("Data"=w589:T1)
          n136 = call-poly "CoreLib.byte array 2 data.vi"("byteArray"=w589) -> ("byteArray out"=w588:T1, "i16"=w586:i16)  [unwired: 16 in, 1 out]
          n137 = call-poly "CoreLib.byte array 2 data.vi"("byteArray"=w588) -> ("byteArray out"=w587:T1, "d64"=w574:dbl)  [unwired: 16 in, 1 out]
          n138 = call-poly "CoreLib.byte array 2 data.vi"("byteArray"=w587) -> ("string"=w591:string)  [unwired: 16 in, 2 out]
          n139 = call "LEBITplc.PenningSetValue.vi"("i ref in"=w583, "Nickname in"=w585, "i attribute in"=w579, "value"=w574, "index in"=w573, "error in"=w581) -> ("In Range?"=w577:bool, "i ref out"=w582:refnum<vi>, "Nicknames out"=w584:string[], "Index out"=w575:i32[], "values"=w578:dbl[], "Log Out?"=w576:bool[], "error out"=w580:errorcluster)  [unwired: 7 in]
          n140 = Type Cast(type=TRUE, x=w591) -> (*(type *) &x=w590:bool)
          n141 = for {
            tunnel: [w614] -> w597
            tunnel: [w613] -> w596
            tunnel: w582 -> [w612]
            tunnel: w580 -> [w611]
            tunnel: w590 -> [w610]
            tunnel: w586 -> [w609]
            tunnel: w584 -> [w608] mode=indexing
            tunnel: w578 -> [w607] mode=indexing
            tunnel: w577 -> [w606]
            tunnel: w576 -> [w605] mode=indexing
            tunnel: w575 -> [w604] mode=indexing
            n142 = case "Command From GUI?" shown="False" w610 {
              selector: w610 -> [_ w631]
              tunnel: [w623 w633] -> w614
              tunnel: [w622 w632] -> w613
              tunnel: w608 -> [w621 w628]
              tunnel: w612 -> [w620 w629]
              tunnel: w611 -> [w619 w627]
              tunnel: w609 -> [w618 w630]
              tunnel: w606 -> [_ w626]
              tunnel: w607 -> [w617 w625]
              tunnel: w605 -> [w616 _]
              tunnel: w604 -> [w615 w624]
              frame True {
                n143 = call "LEBITplc.SetPLC.vi"("i ref in"=w620, "CommandName"=w621, "Binary Selection"=w618, "Value"=w617, "log?"=w616, "error IO"=w619, "index of element"=w615) -> ("i ref out"=w623:refnum<vi>, "error out"=w622:errorcluster)  [unwired: 11 in]
              }
              frame False {
                n144 = case "In Range?" shown="True" w626 {
                  tunnel: [w636 w646] -> w633
                  tunnel: [w637 w645] -> w632
                  tunnel: w627 -> [_ w644]
                  tunnel: w629 -> [w636 w643]
                  tunnel: w628 -> [_ w642]
                  tunnel: w631 -> [_ w640]
                  tunnel: w630 -> [_ w641]
                  tunnel: w625 -> [_ w639]
                  tunnel: w624 -> [_ w638]
                  frame False {
                    n145 = call "CoreLib.my to LV error.vi"("ErrorTypes"=CoreDefs.error_type."can't execute function", "severityLevel"=CoreDefs.error_severity."error") -> ("myErrorCluster"=w637:errorcluster)  [unwired: 16 in, 1 out]
                  }
                  frame True {
                    n146 = call "LEBITplc.SetPLC.vi"("i ref in"=w643, "CommandName"=w642, "Binary Selection"=w641, "Value"=w639, "log?"=w640, "error IO"=w644, "index of element"=w638) -> ("i ref out"=w646:refnum<vi>, "error out"=w645:errorcluster)  [unwired: 11 in]
                  }
                }
              }
            }
          }
          n147 = call "BaseProcess.set event status.vi"("i ref in"=w597, "EventStatus"=w598, "error in (no error)"=w596) -> ("i ref out"=w599:refnum<vi>, "error out"=w600:errorcluster)  [unwired: 14 in, 1 out]
          n148 = case shown="No Error" w600 {
            selector: w600 -> [_ w649]
            tunnel: [_ w648] -> w601
            frame No Error {
            }
            frame Error {
              n149 = Unbundle By Name(w649) -> ("source"=w647:string)
              n150 = call-poly "CoreLib.data 2 byte array.vi"("string"=w647) -> ("byteArray out"=w648:T1)  [unwired: 18 in]
            }
          }
          n151 = Unbundle By Name(w600) -> ("code"=w603:i32)
          n152 = Bundle By Name(cluster=w593, "Data"=w601, "Error #"=w603) -> (w602:T2)
        }
        frame "TrendMsg" {
          # "PLC Value of Monitor"
          # "Get Special"
          # "Get Index of\nMonitor"
          # "Get the Indices of the Monitor \nDependents"
          # "Get Special, Nickname, MonValuePLC and Dependent Monitors"
          n153 = call "CAEObj.unfold trend data.vi"("i ref in"=w676, "raw trend data"=w677, "error in (no error)"=w673) -> ("quality"=w671:i32, "no link"=w670:bool, "i ref out"=w675:refnum<vi>, "data"=w669:i8[], "serviceName"=w668:string, "error out"=w672:errorcluster)  [unwired: 8 in, 3 out]
          n154 = call "LEBITplc.get i attribute.vi"("i ref in"=w675, "error in (no error)"=w672) -> ("i ref out"=w664:refnum<vi>, "i attribute"=w659:T6, "error out"=w665:errorcluster)  [unwired: 15 in]
          n155 = Unbundle By Name(w659) -> ("Special"=w661:string[], "nickNames"=w662:string[], "monValuePLC"=w663:string[], "Dependent-Monitors"=w655:string[][])
          n156 = Search 1D Array(1D array=w663, element=w668) -> (index of element=w650:i32)  [unwired: 1 in]
          n157 = Index Array(array=w662, index=w650) -> (element=w656:string)
          n158 = Index Array(array=w655, index (col)=0 ("disabled index (col)")) -> (element=w658:string[])  [unwired: 1 in]
          n159 = Search 1D Array(1D array=w658, element=w656) -> (index of element=w654:i32)  [unwired: 1 in]
          n160 = Index Array(array=w655, index (row)=w654) -> (element=w653:string[])  [unwired: 1 in]
          n161 = Delete From Array(array=w653, index=0) -> (array with subset deleted=w651:string[])  [unwired: 1 in, 1 out]
          n162 = Index Array(array=w661, index=w650) -> (element=w660:string)
          n163 = case "Deal with Special Monitors" shown="Default" w660 {
            tunnel: w665 -> [w695 w716 w740 w764]
            tunnel: w671 -> [w679 w721 w745 w769]
            tunnel: w670 -> [w682 w710 w734 w758]
            tunnel: [w683 w708 w732 w756] -> w666
            tunnel: w664 -> [w694 w720 w744 w768]
            tunnel: w669 -> [w691 w719 w743 w767]
            tunnel: w659 -> [w693 w718 w742 w766]
            tunnel: w650 -> [w689 w717 w741 w765]
            tunnel: w656 -> [_ w715 w739 w763]
            tunnel: [w681 w709 w733 w757] -> w667
            tunnel: w651 -> [w678 _ _ _]
            frame Default {
              # "Set Monitor Dependents to the Currently\nAcquired Monitor Values"
              # "Normal Monitor Values"
              n164 = Array Size(array=w678) -> (size(s)=w686:i32)
              n165 = Type Cast(type=0.0, x=w691) -> (*(type *) &x=w692:dbl)
              n166 = Not Equal To 0?(x=w686) -> (x != 0?=w685:bool)
              n167 = call "LEBITplc.TrendMessage.vi"("i ref in"=w694, "data"=w692, "i attribute"=w693, "index"=w689, "error in"=w695, "quality"=w679, "no link"=w682) -> ("i ref out"=w688:refnum<vi>, "data out"=w680:dbl, "i attribute out"=w684:T6, "error out"=w687:errorcluster)  [unwired: 9 in]
              n168 = case "Has Monitor Dependents" shown="True" w685 {
                tunnel: w688 -> [w697 w704]
                tunnel: w687 -> [w696 w702]
                tunnel: w684 -> [_ w705]
                tunnel: [w697 w700] -> w683
                tunnel: [w696 w701] -> w681
                tunnel: w682 -> [_ w706]
                tunnel: w678 -> [_ w703]
                tunnel: w680 -> [_ w699]
                tunnel: w679 -> [_ w698]
                frame False {
                }
                frame True {
                  n169 = call "LEBITplc.UpdateMonDep.vi"("i ref in"=w704, "data"=w699, "i attribute"=w705, "DependentMonitors"=w703, "error in"=w702, "quality"=w698, "no link"=w706) -> ("i ref out"=w700:refnum<vi>, "error out"=w701:errorcluster)  [unwired: 10 in, 1 out]
                }
              }
            }
            frame "IonGuide" {
              # "Deal With Special IonGuide Monitor Values"
              n170 = call "LEBITplc.IGMonitor.vi"("i ref in"=w720, "data"=w719, "i attribute in"=w718, "index"=w717, "NickNames"=w715, "error in"=w716, "no link"=w710) -> ("i ref out"=w714:refnum<vi>, "Data"=w707:dbl[], "i attribute out"=w713:T6, "Indexs"=w712:i32[], "error out"=w711:errorcluster)  [unwired: 8 in]
              n171 = for "For All Monitor Values" {
                tunnel: [w730] -> w709
                tunnel: w721 -> [w729]
                tunnel: w710 -> [w728]
                tunnel: w713 -> [w726]
                tunnel: w712 -> [w723] mode=indexing
                tunnel: w711 -> [w725]
                tunnel: w707 -> [w722] mode=indexing
                shift-right: [w724] -> w708
                shift-left: w714 -> [w727]
                n172 = call "LEBITplc.TrendMessage.vi"("i ref in"=w727, "data"=w722, "i attribute"=w726, "index"=w723, "error in"=w725, "quality"=w729, "no link"=w728) -> ("i ref out"=w724:refnum<vi>, "error out"=w730:errorcluster)  [unwired: 9 in, 2 out]
              }
            }
            frame "TestIonSource" {
              # "Deal With Special IonGuide Monitor Values"
              n173 = call "LEBITplc.TestIonSourceMonitor.vi"("i ref in"=w744, "data"=w743, "i attribute in"=w742, "index"=w741, "NickNames"=w739, "error in"=w740, "no link"=w734) -> ("i ref out"=w738:refnum<vi>, "Data"=w731:dbl[], "i attribute out"=w737:T6, "Indexs"=w736:i32[], "error out"=w735:errorcluster)  [unwired: 8 in]
              n174 = for "For All Monitor Values" {
                tunnel: [w754] -> w733
                tunnel: w745 -> [w753]
                tunnel: w734 -> [w752]
                tunnel: w737 -> [w751]
                tunnel: w731 -> [w746] mode=indexing
                tunnel: w736 -> [w748] mode=indexing
                tunnel: w735 -> [w750]
                shift-right: [w749] -> w732
                shift-left: w738 -> [w747]
                n175 = call "LEBITplc.TrendMessage.vi"("i ref in"=w747, "data"=w746, "i attribute"=w751, "index"=w748, "error in"=w750, "quality"=w753, "no link"=w752) -> ("i ref out"=w749:refnum<vi>, "error out"=w754:errorcluster)  [unwired: 9 in, 2 out]
              }
            }
            frame "Bob1toBun" {
              # "Deal With Special Bob1toBun Monitor Values"
              n176 = call "LEBITplc.Bob1toBunMonitor.vi"("i ref in"=w768, "data"=w767, "i attribute in"=w766, "index"=w765, "NickNames"=w763, "error in"=w764, "no link"=w758) -> ("i ref out"=w762:refnum<vi>, "Data"=w755:dbl[], "i attribute out"=w761:T6, "Indexs"=w760:i32[], "error out"=w759:errorcluster)  [unwired: 8 in]
              n177 = for "For All Monitor Values" {
                tunnel: [w778] -> w757
                tunnel: w769 -> [w777]
                tunnel: w758 -> [w776]
                tunnel: w761 -> [w774]
                tunnel: w760 -> [w771] mode=indexing
                tunnel: w759 -> [w773]
                shift-right: [w772] -> w756
                shift-left: w762 -> [w775]
                tunnel: w755 -> [w770] mode=indexing
                n178 = call "LEBITplc.TrendMessage.vi"("i ref in"=w775, "data"=w770, "i attribute"=w774, "index"=w771, "error in"=w773, "quality"=w777, "no link"=w776) -> ("i ref out"=w772:refnum<vi>, "error out"=w778:errorcluster)  [unwired: 9 in, 2 out]
              }
            }
          }
        }
        frame "UpdateLLF" {
          # "LoadOrSave?"
          # "Log?"
          # "Log"
          # "File-Name"
          # "GUI-Name"
          n179 = Unbundle By Name(w802) -> ("Data"=w804:T1)
          n180 = call-poly "CoreLib.byte array 2 data.vi"("byteArray"=w804, "error in (no error)"=w799) -> ("byteArray out"=w796:T1, "string"=w784:string, "error out"=w794:errorcluster)  [unwired: 15 in]
          n181 = call-poly "CoreLib.byte array 2 data.vi"("byteArray"=w796, "error in (no error)"=w794) -> ("byteArray out"=w785:T1, "string"=w795:string, "error out"=w786:errorcluster)  [unwired: 15 in]
          n182 = call-poly "CoreLib.byte array 2 data.vi"("byteArray"=w785, "error in (no error)"=w786) -> ("byteArray out"=w782:T1, "string"=w787:string, "error out"=w783:errorcluster)  [unwired: 15 in]
          n183 = Type Cast(type=TRUE, x=w787) -> (*(type *) &x=w780:bool)
          n184 = call-poly "CoreLib.byte array 2 data.vi"("byteArray"=w782, "error in (no error)"=w783) -> ("i16"=w779:i16, "error out"=w781:errorcluster)  [unwired: 15 in, 1 out]
          n185 = call "LEBITplc.GetLastLoadedLocation.vi"("i ref in"=w793, "error in (no error)"=w781) -> ("i ref out"=w792:refnum<vi>, "LLFLocation"=w789:string, "error out"=w791:errorcluster)  [unwired: 15 in]
          n186 = String To Path(string=w789) -> (path=w790:path)
          n187 = call "LEBITplc.UpdateLLF.vi"("i ref in"=w792, "file path (use dialog)"=w790, "FileName"=w795, "GUI Name"=w784, "error in"=w791, "LoadorSave"=w779, "Log"=w780) -> ("i ref in"=w798:refnum<vi>, "error out"=w797:errorcluster)  [unwired: 11 in]
          n188 = case shown="No Error" w797 {
            selector: w797 -> [_ w807]
            tunnel: [_ w806] -> w800
            frame No Error {
            }
            frame Error {
              n189 = Unbundle By Name(w807) -> ("source"=w805:string)
              n190 = call-poly "CoreLib.data 2 byte array.vi"("string"=w805) -> ("byteArray out"=w806:T1)  [unwired: 18 in]
            }
          }
          n191 = Unbundle By Name(w797) -> ("code"=w801:i32)
          n192 = Bundle By Name(cluster=w802, "Data"=w800, "Error #"=w801) -> (w803:T2)
        }
      }
    }
    frame Error {
    }
  }
  "answer cluster" <- w13
  "i ref out" <- w10
  "error out" <- w9
